vi "setUserEvent.vi"(8 "error in (no error)":errorcluster, 11 "ForecastDisplay in":refnum<class "ForecastDisplay.lvclass">) -> (0 "error out":errorcluster, 3 "ForecastDisplay out":refnum<class "ForecastDisplay.lvclass">)   [LabVIEW 2017, in "ForecastDisplay.lvclass"]
uses:
  ForecastDisplay.lvclass
  Observer/Observer.lvclass
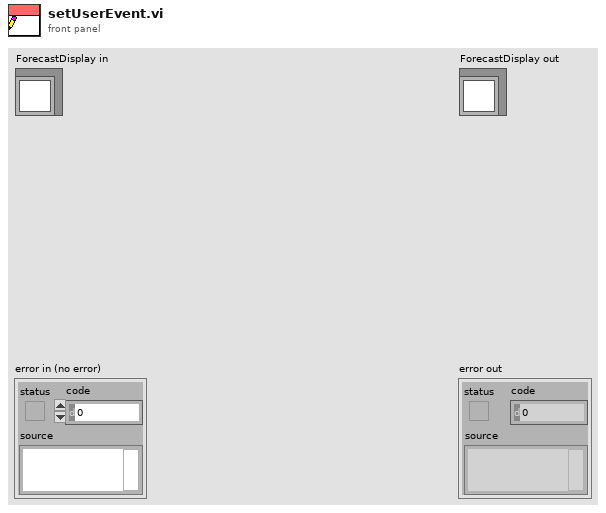
[diagram p1: front panel]
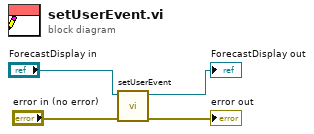
[diagram p0: block diagram]
diagram:
  n1 = call-parent "setUserEvent.vi"("error in (no error)"="error in (no error)", "Observer in"="ForecastDisplay in") -> ("error out"=→"error out":errorcluster, "Observer out"=→"ForecastDisplay out":refnum<class "ForecastDisplay.lvclass">)  [unwired: 8 in]
